vi "DAQmx Create Channel (CI-Position-Linear Encoder).vi"(0 "task in":refnum<k21>, 1 "z index enable":bool, 2 "z index value":dbl, 3 "z index phase":i32(ring)=10040 items=["A High B High"=10040, "A High B Low"=10041, "A Low B High"=10042, "A Low B Low"=10043], 5 "counter":tag, 6 "decoding type":i32(ring)=10092 items=["X1"=10090, "X2"=10091, "X4"=10092, "Two Pulse Counting"=10313], 7 "name to assign":string, 9 "units":i32(ring)=10219 items=["Meters"=10219, "Inches"=10379, "Ticks"=10304, "From Custom Scale"=10065], 11 "error in":errorcluster, 12 "custom scale name":tag, 13 "distance per pulse":dbl=0.001, 14 "initial position":dbl) -> (4 "task out":refnum<k21>, 15 "error out":errorcluster)   [LabVIEW 2018]
doc: "Creates a channel that uses a linear encoder to measure linear position. With the exception of devices that support multi-counter tasks, you can create only one counter input channel at a time with this VI because a task can contain only one counter input channel. To read from multiple counters simultaneously, use a separate task for each counter. Connect the input signals to the default input terminals of the counter unless you select different input terminals."
uses:
  nilvaiu.dll
panel:
  # "z index info"
  # "encoder info"
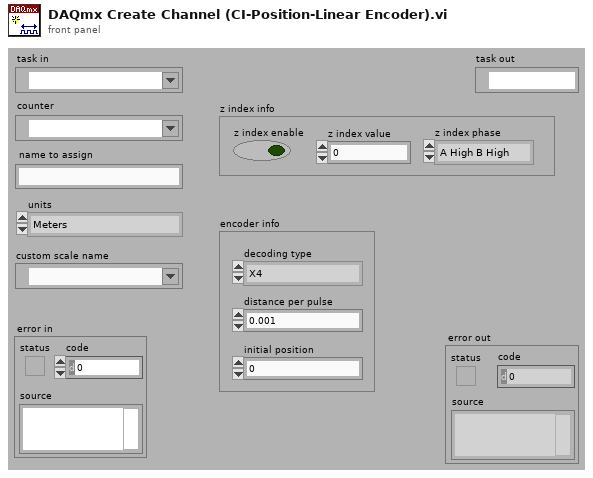
[diagram p1: front panel]
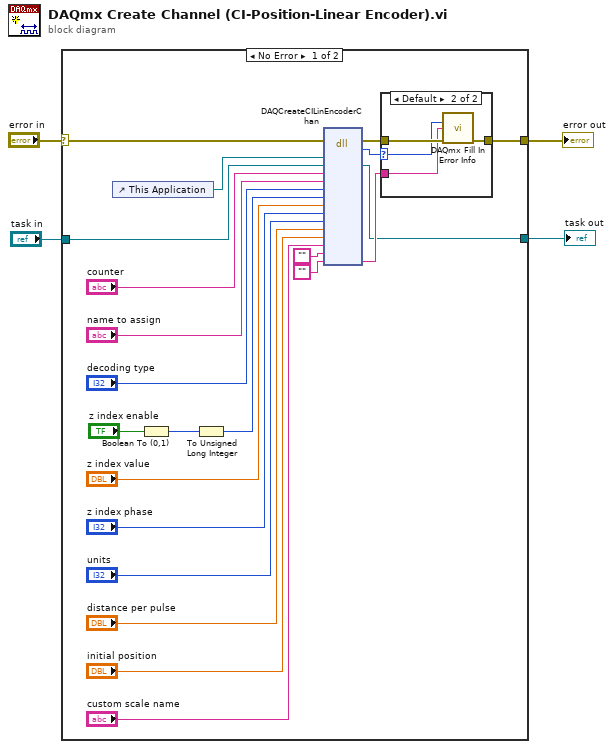
[diagram p0: block diagram]
diagram:
  n1 = case shown="No Error" "error in" {
    selector: "error in" -> [w6 w33]
    tunnel: [w21 w33] -> w4
    tunnel: [w20 w32] -> w3
    tunnel: "task in" -> [w10 w32]
    frame No Error {
      n2 = control-ref of="This Application"() -> (w23:refnum<vi>)
      n3 = Boolean To (0,1)(Boolean="z index enable") -> (0, 1=w8:i16)
      n4 = To Unsigned Long Integer(number=w8) -> (unsigned 32bit integer=w7:u32)
      n5 = dll-call lib="nilvaiu.*" fn="DAQCreateCILinEncoderChan"(error in=w6, "lvAppRef"=w23, "refObjPtr"=w10, "counter"="counter", "channelNameIn"="name to assign", "decodingType"="decoding type", "ZidxEnable"=w7, "ZidxVal"="z index value", "ZidsPhase"="z index phase", "units"="units", "distPerPulse"="distance per pulse", "initialPos"="initial position", "customScaleName"="custom scale name", "channelNamesOut"="", "extendedErrorInfo"="") -> (error out=w26:errorcluster, "return type"=w25:i32, "refObjPtr"=w20:refnum<k21>, "extendedErrorInfo"=w24:string)  [unwired: 14 in, 1 out]
      n6 = case shown="Default" w25 {
        selector: w25 -> [_ w29]
        tunnel: w26 -> [w27 w31]
        tunnel: [w27 w30] -> w21
        tunnel: w24 -> [_ w28]
        frame 0 {
        }
        frame Default {
          n7 = call "DAQmx Fill In Error Info.vi"("status code"=w29, "extended error info"=w28, "error in"=w31) -> ("error out"=w30:errorcluster)  [unwired: 1 in, 11 out]
        }
      }
    }
    frame Error {
    }
  }
  "error out" <- w4
  "task out" <- w3
